vi "Write Tare Settings.vi"(7 "Unit ID (A)":string="A", 8 "error in":errorcluster, 10 "Tare Functions":T1={"Display"=enum."None", "External"=enum."None", "Auto-Tare Delay [s]"=nan} {"Auto-Tare Delay [s]" min=0.0 max=25.5 step=0.1 format="%.1g"}, 11 "VISA Session In":refnum<visa-resource-name>="Alicat") -> (0 "error out":errorcluster, 3 "VISA Session Out":refnum<visa-resource-name>)   [LabVIEW 2014]
doc: "Writes the tare options to an Alicat device: variable associated with the front panel tare button, variable associated with the remote tare pin (only applicable for meters), and the auto tare delay upon power up (a 0 indicates that no tare is performed on power up)."
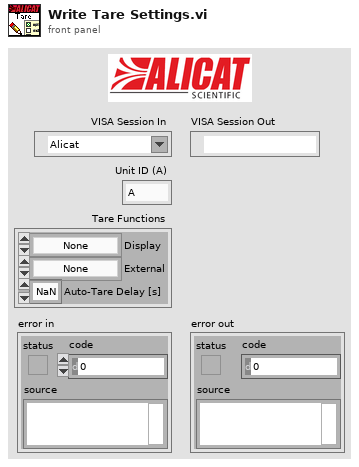
[diagram p1: front panel]
types:
  T1 = cluster{"Display":enum16{"None", "Pressure", "Volumetric"}, "External":enum16{"None", "Pressure", "Volumetric", "Totalizer"}, "Auto-Tare Delay [s]":dbl}
  T2 = enum16{"None", "Pressure", "Volumetric", "Totalizer"}
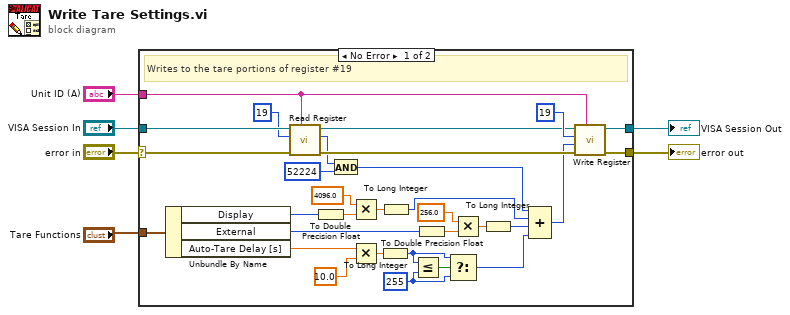
[diagram p0: block diagram]
diagram:
  n1 = case shown="No Error" "error in" {
    selector: "error in" -> [w7 w38]
    tunnel: [w37 w39] -> w6
    tunnel: [w36 w38] -> w5
    tunnel: "Tare Functions" -> [w34 _]
    tunnel: "VISA Session In" -> [w16 w39]
    tunnel: "Unit ID (A)" -> [w13 _]
    frame No Error {
      w29 = 255 ("y")
      # "Writes to the tare portions of register #19"
      n2 = Unbundle By Name(w34) -> ("Display"=w27:enum16{"None", "Pressure", "Volumetric"}, "External"=w20:T2, "Auto-Tare Delay [s]"=w33:dbl)
      n3 = call "Read Register.vi"("Unit ID (A)"=w13, "error in"=w7, "Register address"=u16 19, "VISA Session In"=w16) -> ("error out"=w15:errorcluster, "Register Value (I32)"=w11:i32, "VISA Session Out"=w14:refnum<visa-resource-name>)  [unwired: 5 in]
      n4 = To Double Precision Float(number=w27) -> (double precision float=w26:dbl)
      n5 = And(x=w11, y=52224 ("32bit integer")) -> (x .and. y?=w9:i32)
      n6 = Multiply(x=4096.0, y=w26) -> (x*y=w24:dbl)
      n7 = Multiply(x=w33, y=10.0) -> (x*y=w31:dbl)
      n8 = To Long Integer(number=w31) -> (32bit integer=w28:i32)
      n9 = To Long Integer(number=w24) -> (32bit integer=w19:i32)
      n10 = Less Or Equal?(x=w28, y=w29) -> (x <= y?=w30:bool)
      n11 = To Double Precision Float(number=w20) -> (double precision float=w21:dbl)
      n12 = Select(t=w28, s=w30, f=w29) -> (s? t:f=w17:i32)
      n13 = Multiply(x=256.0, y=w21) -> (x*y=w23:dbl)
      n14 = To Long Integer(number=w23) -> (32bit integer=w18:i32)
      n15 = Compound Arithmetic op=ADD(w9, w19, w18, w17) -> (w8:i32)
      n16 = call "Write Register.vi"("Unit ID (A)"=w13, "error in"=w15, "Register Value"=w8, "Register address"=u16 19, "VISA Session In"=w14) -> ("error out"=w36:errorcluster, "VISA Session Out"=w37:refnum<visa-resource-name>)  [unwired: 4 in, 1 out]
    }
    frame Error {
    }
  }
  "error out" <- w5
  "VISA Session Out" <- w6
